vi "Get Description.vi"(8 "error in":errorcluster, 11 "Lv Proj Document Type:TAF Proj":refnum<class "TAF Proj.lvclass">) -> (0 "error out":errorcluster, 2 "Description":string, 3 "Name":string)   [LabVIEW 2021, in "TAF Proj Document Type.lvlib" / "TAF Proj.lvclass"]
doc: "Overide this function to define the name of the document type and give a description of its goal.\n\nNote: These inforamtion are used to help user to select the correct document type."
uses:
  <vilib>/Wovalab/AntiDoc/Document Type/Add-ons/LabVIEW TAF Project/TAF Proj/TAF Proj.lvclass
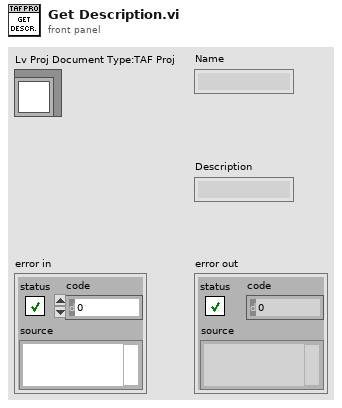
[diagram p1: front panel]
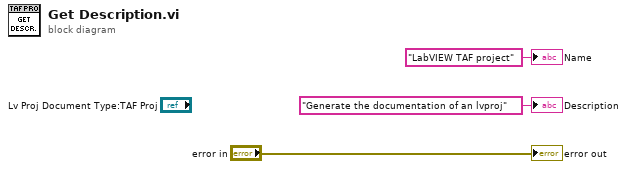
[diagram p0: block diagram]
diagram:
  "error out" <- "error in"
  "Name" <- "LabVIEW TAF project" ("Name")
  "Description" <- "Generate the documentation of an lvproj" ("Description")
